vi "DaemonShutdown.vi"(8 "error in (no error)":errorcluster, 11 "queue cluster":T1) -> (0 "error out":errorcluster, 3 "queue cluster out":T1)   [LabVIEW 2014]
uses:
  typedefs/clientStatus.ctl
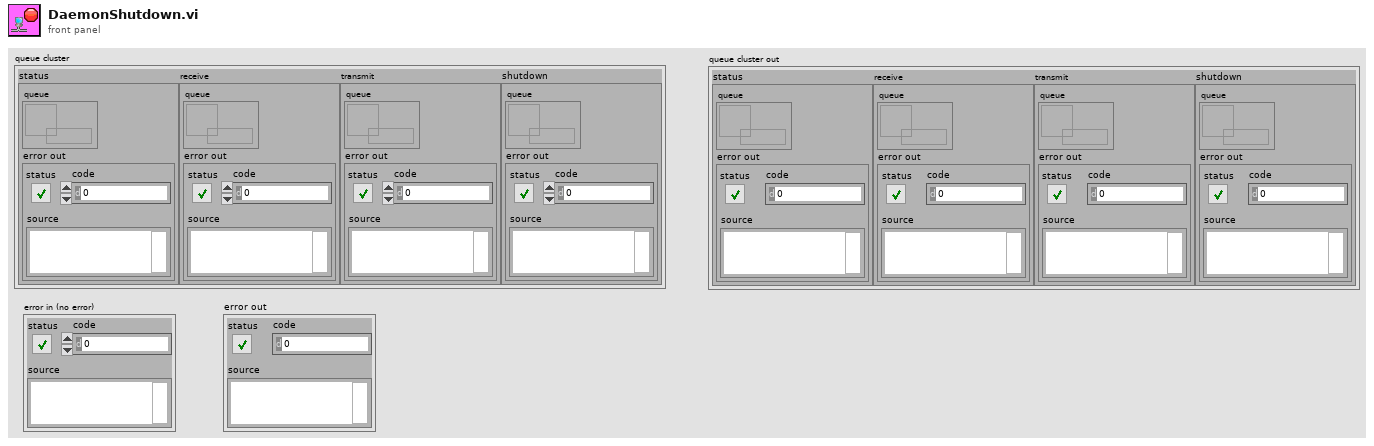
[diagram p1: front panel]
types:
  T1 = cluster{"status":cluster{"queue":refnum<queue>, "error out":errorcluster}, "receive":cluster{"queue":refnum<queue>, "error out":errorcluster}, "transmit":cluster{"queue":refnum<queue>, "error out":errorcluster}, "shutdown":cluster{"queue":refnum<queue>, "error out":errorcluster}}
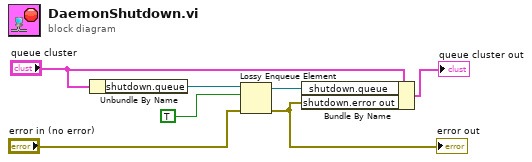
[diagram p0: block diagram]
diagram:
  n1 = Unbundle By Name("queue cluster") -> ("shutdown.queue"=w7:refnum<queue>)
  n2 = Lossy Enqueue Element(queue=w7, element=TRUE, error in (no error)="error in (no error)") -> (queue out=w2:refnum<queue>, error out=w3:errorcluster)  [unwired: 2 out]
  "error out" <- w3
  n3 = Bundle By Name(cluster="queue cluster", "shutdown.queue"=w2, "shutdown.error out"=w3) -> (→"queue cluster out":T1)
